vi "mainPrint.vi"(8 "Error In":errorcluster, 11 "printUDE":T1) -> (0 "Error Out":errorcluster)   [LabVIEW 2018]
uses:
  controls/printUDE.ctl
  controls/printData.ctl
  controls/serialPortEnum.ctl
panel:
  out "Boolean":bool
  in  "Print":bool
  in  "Stop":bool
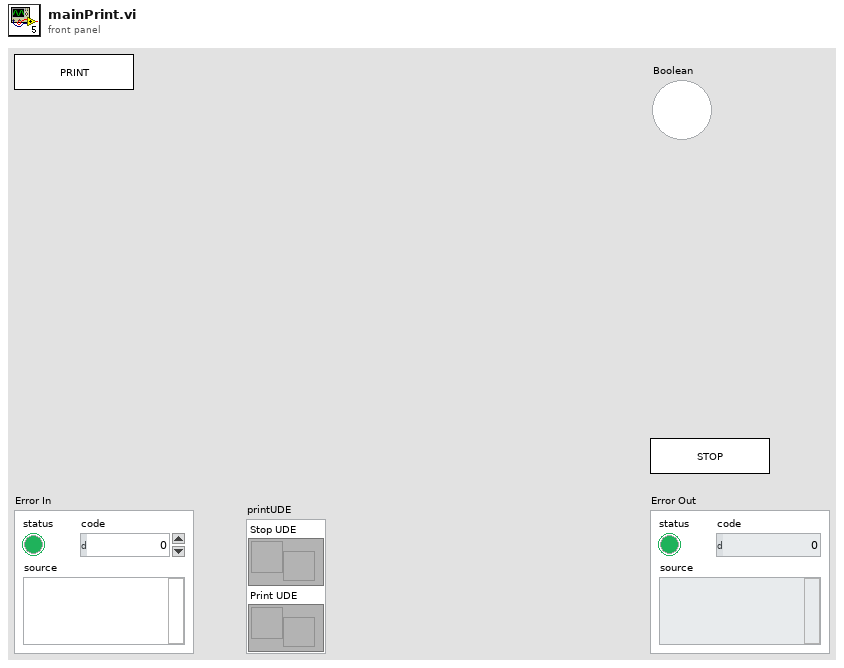
[diagram p1: front panel]
types:
  T1 = typedef "printUDE.ctl" = cluster{"Stop UDE":refnum<user-event>, "Print UDE":refnum<user-event>}
  T2 = enum32{"Invalid", "Standard", "Closed", "Hidden", "Minimized", "Maximized"}
  T3 = enum32{"invalid app kind", "Development System", "Run Time System", "Student Edition", "Embedded LabVIEW", "Evaluation", "Custom"}
  T4 = typedef "serialPortEnum.ctl" = enum16{"init", "write", "read", "close"}
  T5 = typedef "printData.ctl" = cluster{"Print Button":bool, "VISA resource name":refnum<visa-resource-name>, "Status?":bool, "Scan?":bool}
  T6 = cluster{"Core":cluster{"Current VI Reference":refnum<vi>, "Close Panel on Exit?":bool}, "printUDE":T1, "Print Data":T5, "QR":string, "Status":bool, "comPort":refnum<visa-resource-name>}
  T7 = cluster{"Current VI Reference":refnum<vi>, "Close Panel on Exit?":bool}
  T8 = typedef "pathCluster.ctl" = cluster{"src Folder Path":path, "Controller Module Path":path, "UI Module Path":path, "Model Select Module Path":path, "Barcode Printer Module Path":path, "Barcode Scanner Module Path":path, "Database Module Path":path, "Report Generation Path":path, "Simulation Path":path, "subVIs Folder Path":path, "info Folder Path":path, "config file Path":path, "cutomerLogo Path":path}
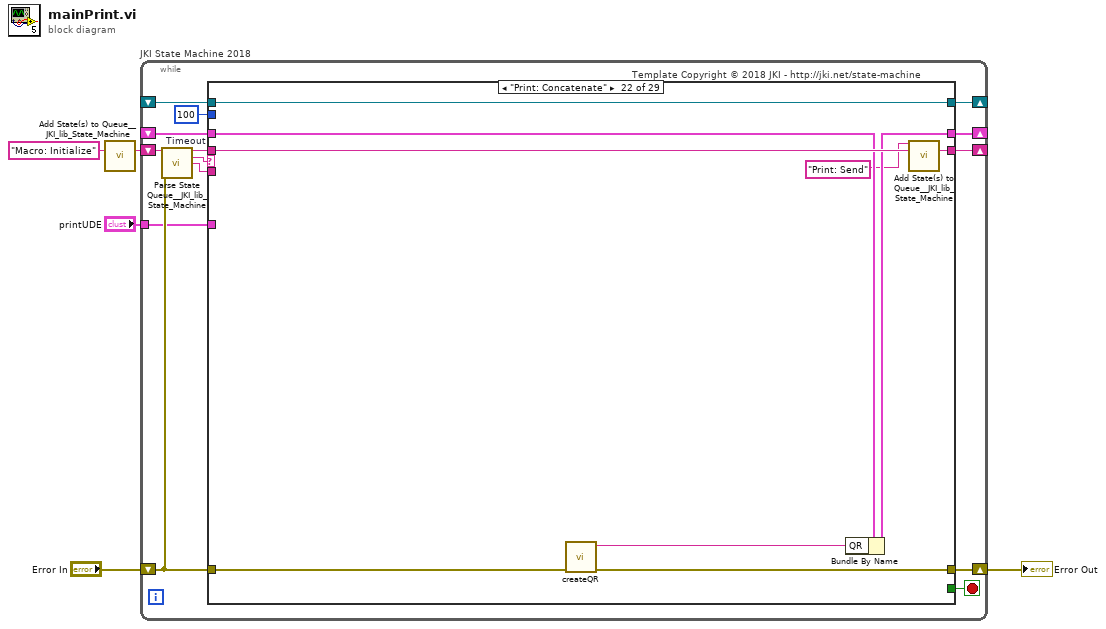
[diagram p0: block diagram]
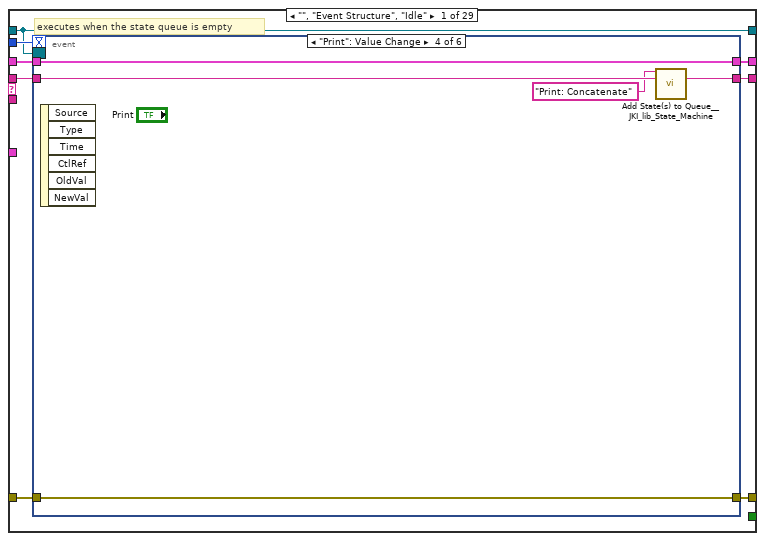
[diagram p2: hidden frame]
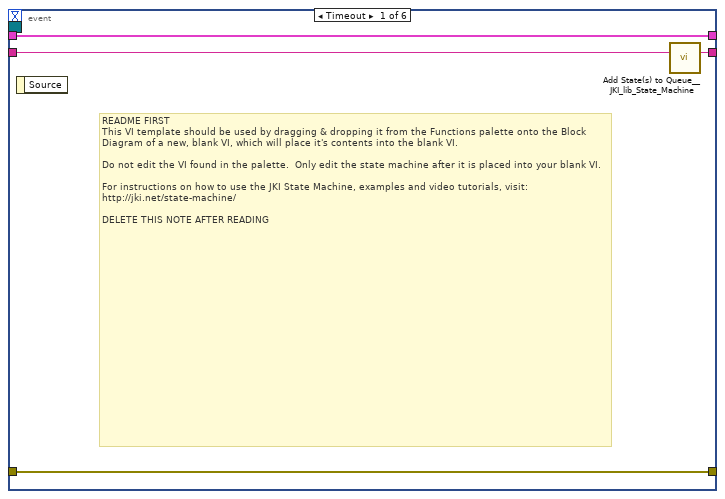
[diagram p3: hidden frame]
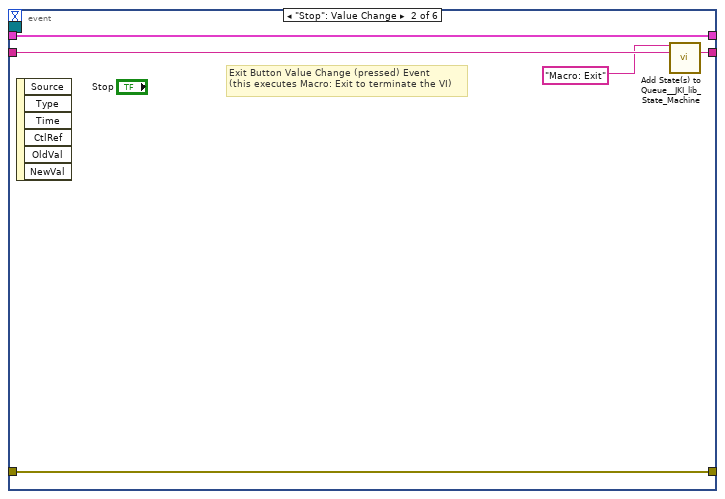
[diagram p4: hidden frame]
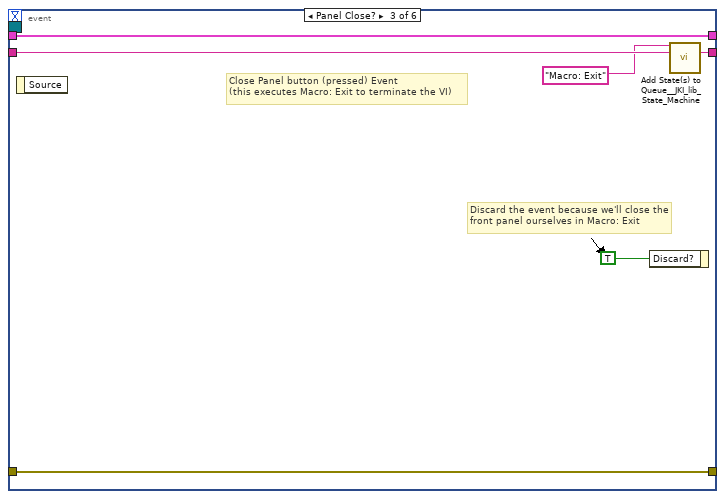
[diagram p5: hidden frame]
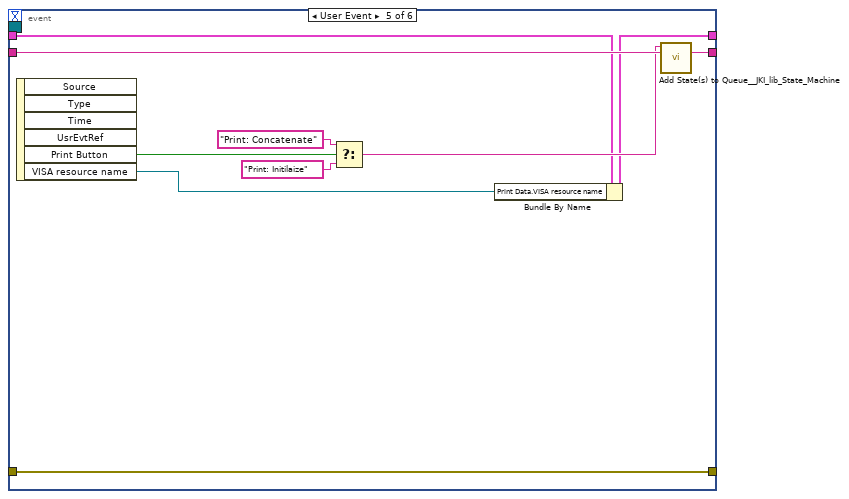
[diagram p6: hidden frame]
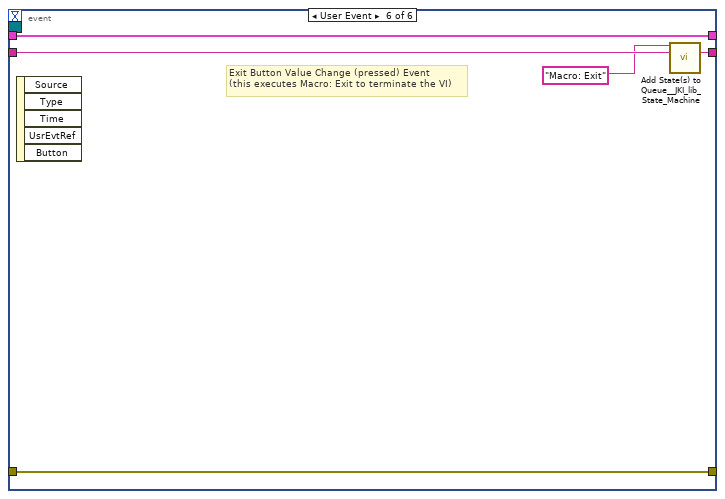
[diagram p7: hidden frame]
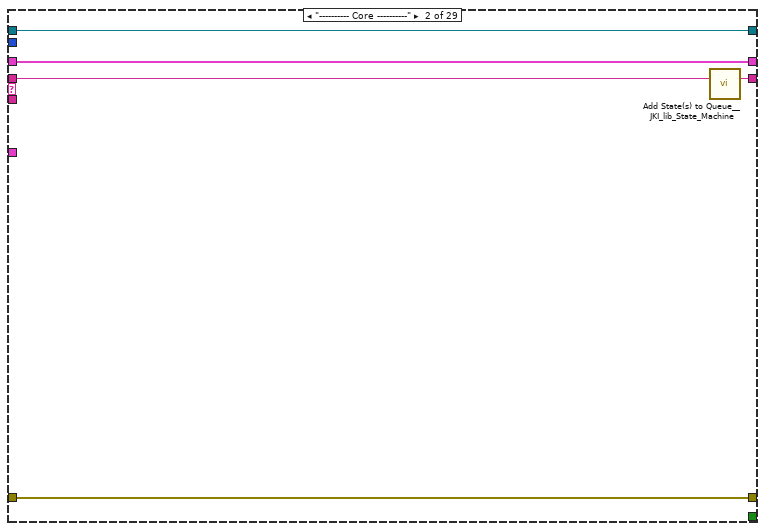
[diagram p8: hidden frame]
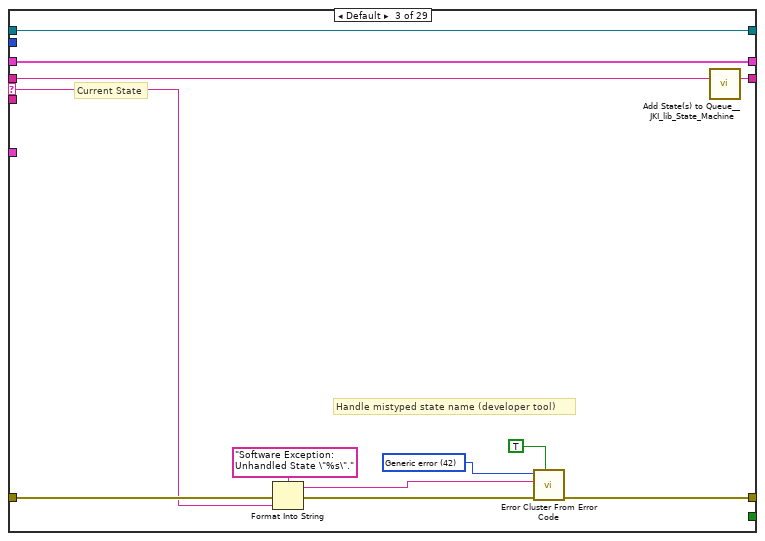
[diagram p9: hidden frame]
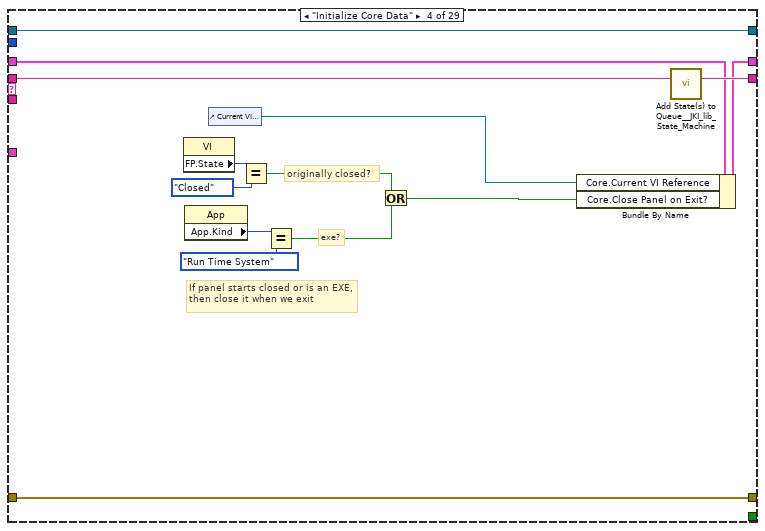
[diagram p10: hidden frame]
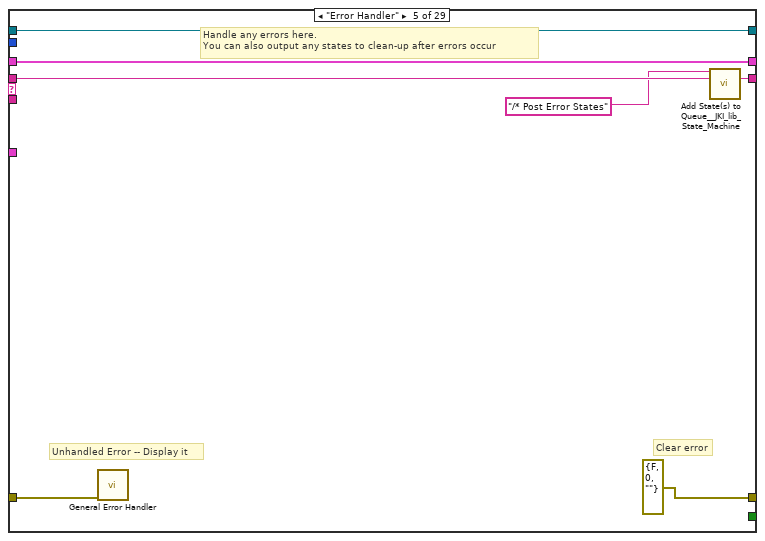
[diagram p11: hidden frame]
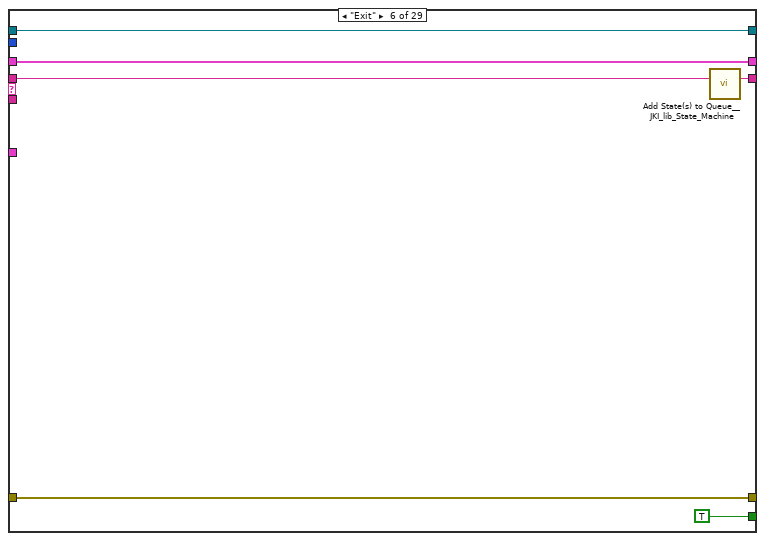
[diagram p12: hidden frame]
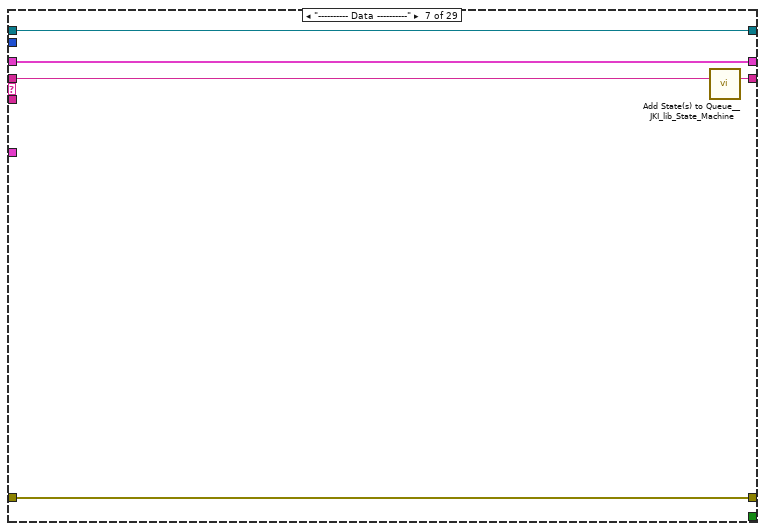
[diagram p13: hidden frame]
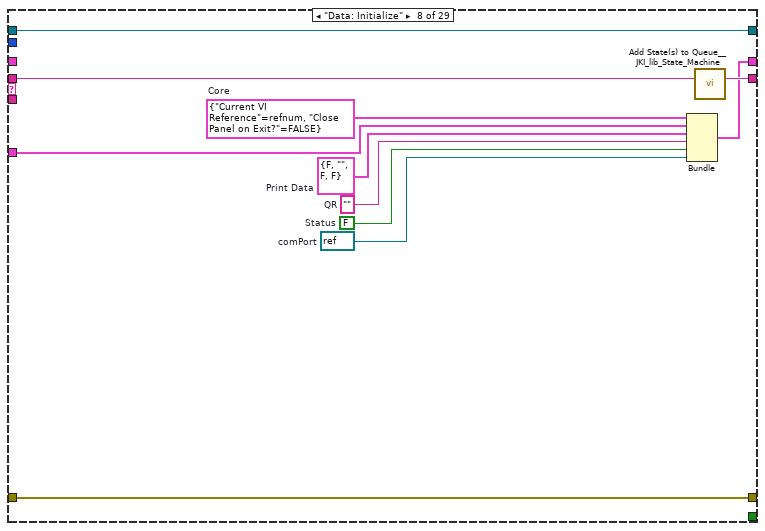
[diagram p14: hidden frame]
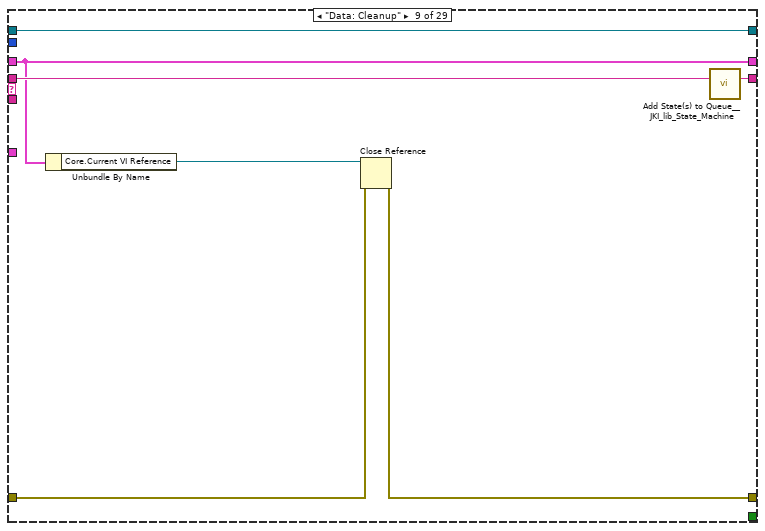
[diagram p15: hidden frame]
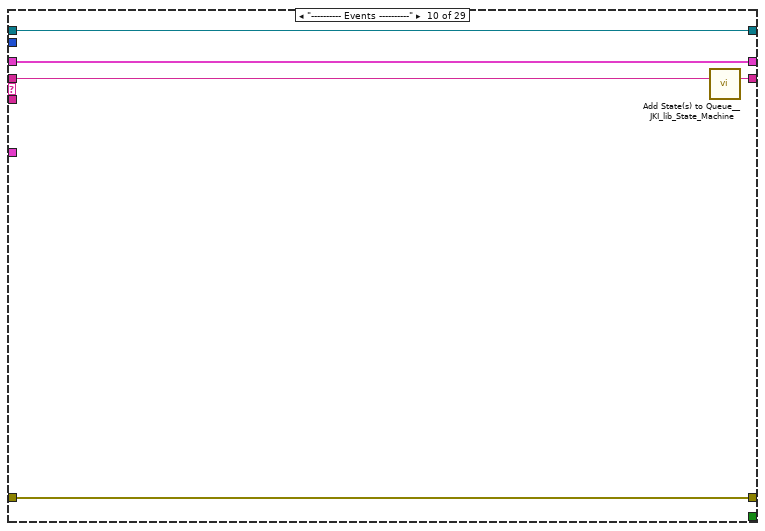
[diagram p16: hidden frame]
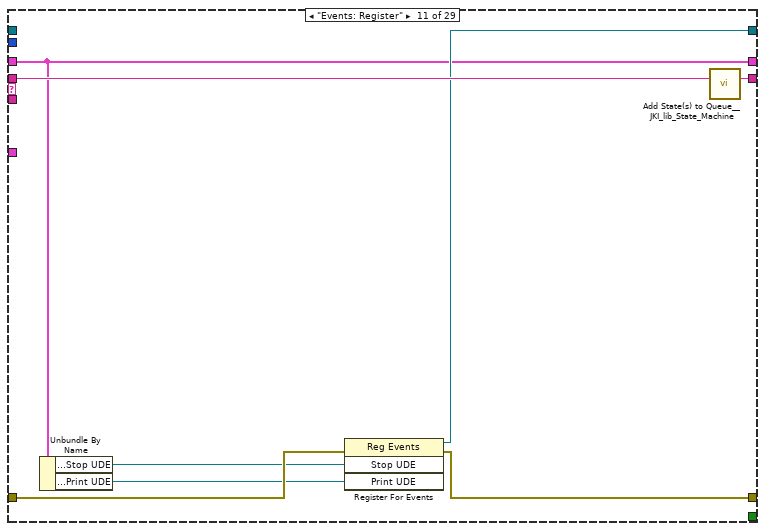
[diagram p17: hidden frame]
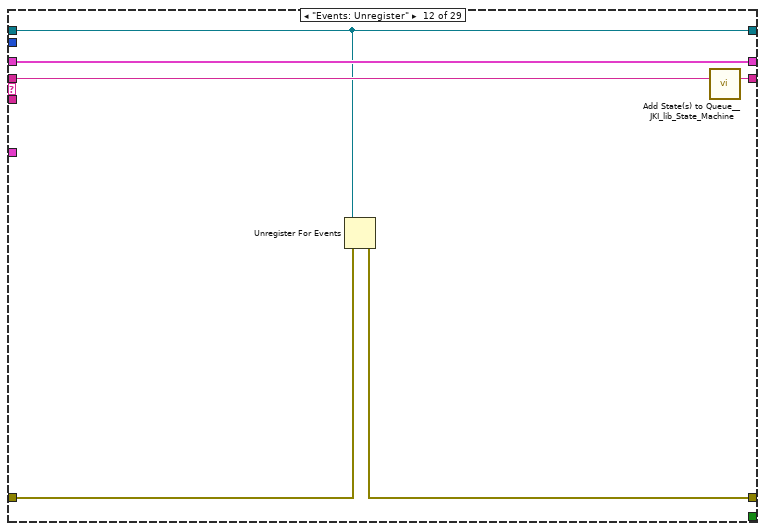
[diagram p18: hidden frame]
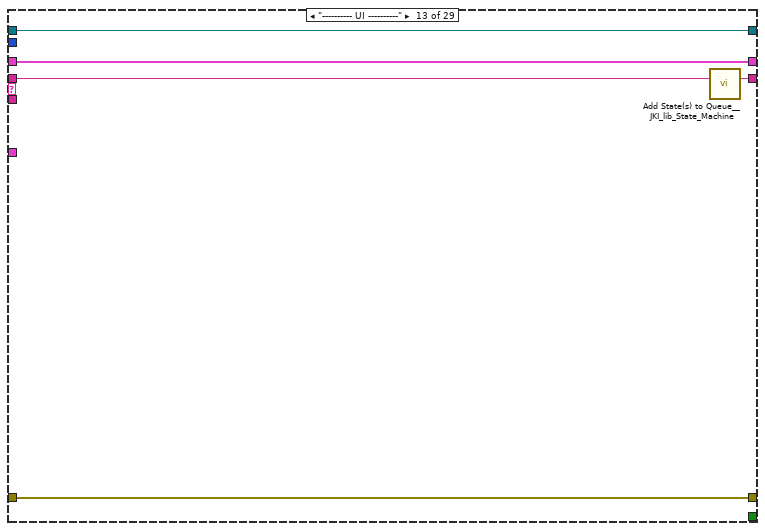
[diagram p19: hidden frame]
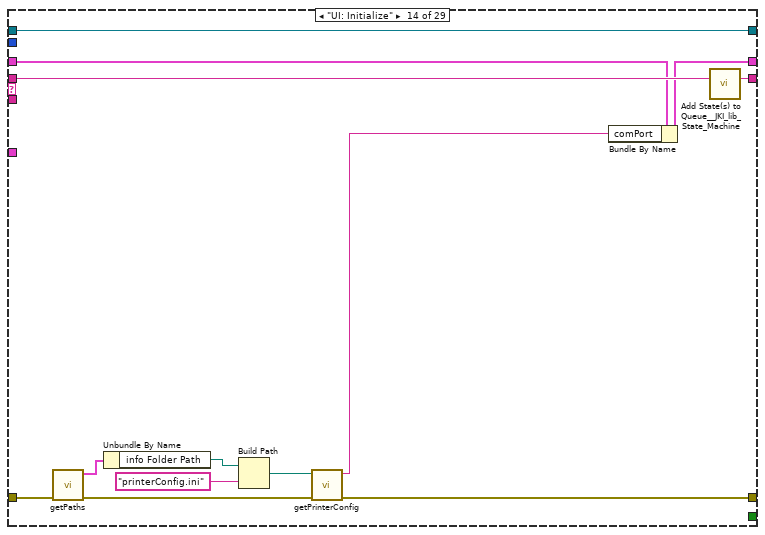
[diagram p20: hidden frame]
diagram:
  n1 = call <vilib>:"Add State(s) to Queue__JKI_lib_State_Machine.vi"("State(s) in (\"\")"="Macro: Initialize") -> ("States Out"=w5:string)  [unwired: 14 in]
  n2 = while "JKI State Machine 2018" {
    shift-right: [w12] -> _
    shift-left: _ -> [w11]
    shift-right: [w15] -> w3
    shift-left: "Error In" -> [w9]
    shift-right: [w14] -> _
    shift-left: w5 -> [w16]
    shift-right: [w8] -> _
    shift-left: _ -> [w7]
    tunnel: "printUDE" -> [w6]
    stop <- w13 stop-if-true
    w10 = 100  # Timeout
    # "Template Copyright © 2018 JKI - http://jki.net/state-machine"
    n3 = call <vilib>:"Parse State Queue__JKI_lib_State_Machine.vi"("State Queue"=w16, "Error In (no error)"=w9) -> ("Remaining States"=w18:string, "Current State"=w19:string, "Arguments"=w17:string)  [unwired: 11 in]
    n4 = case shown="\"Print: Concatenate\"" w19 {
      selector: w19 -> [_ _ w69 _ _ _ _ _ _ _ _ _ _ _ _ _ _ _ _ _ _ _ _ _ _ _ _ _ _]
      tunnel: w18 -> [w27 w67 w73 w93 w100 w106 w111 w122 w129 w134 w142 w148 w153 w166 w173 w185 w255 w261 w272 w277 w288 w297 w309 w316 w321 w333 w346 w351 w357]
      tunnel: w17 -> [_ _ _ _ _ _ _ _ _ _ _ _ _ _ w168 w179 _ _ _ _ _ _ _ _ _ _ _ _ _]
      tunnel: w11 -> [w25 w64 w71 w86 w97 w104 w108 _ w124 w131 w137 w146 w150 w156 w171 w181 w252 w258 w269 w274 w282 w292 w302 w314 w318 w324 w338 w348 w353]
      tunnel: [w24 w65 w75 w90 errorcluster {"status"=FALSE, "code"=0, "source"=""} ("error out") w103 w109 w119 w125 w132 w139 w143 w151 w158 w169 w182 w253 w259 w270 w275 w280 w293 w300 w311 w319 w329 w342 w349 w355] -> w15
      tunnel: w9 -> [w23 w65 w74 w90 w96 w103 w109 w119 w126 w132 w138 w144 w151 w163 w170 w183 w253 w259 w270 w275 w285 w294 w306 w312 w319 w330 w343 w349 w355]
      tunnel: [w26 w66 w72 w92 w99 w105 w110 w121 w128 w133 w141 w147 w152 w165 w172 w184 w254 w260 w271 w276 w287 w296 w308 w315 w320 w332 w345 w350 w356] -> w14
      tunnel: [_ _ _ _ _ TRUE _ _ _ _ _ _ _ _ _ _ _ _ _ _ _ _ _ _ _ _ _ _ _] -> w13
      tunnel: [w22 w64 w71 w91 w97 w104 w108 w120 w124 w131 w137 w146 w150 w155 w171 w181 w252 w258 w269 w274 w281 w291 w301 w314 w318 w323 w337 w348 w353] -> w12
      tunnel: w10 -> [w21 _ _ _ _ _ _ _ _ _ _ _ _ _ _ _ _ _ _ _ _ _ _ _ _ _ _ _ _]
      tunnel: [w20 w63 w68 w80 w94 w101 w107 w117 w123 w130 w140 w145 w149 w164 w167 w178 w251 w256 w262 w273 w286 w295 w307 w313 w317 w331 w344 w347 w354] -> w8
      tunnel: w7 -> [w20 w63 w68 w80 w94 w101 w107 w117 w123 w130 _ w145 w149 w164 w167 w178 w251 w256 w262 w273 w286 w295 w307 w313 w317 w331 w344 w347 w354]
      tunnel: w6 -> [_ _ _ _ _ _ _ w116 _ _ _ _ _ _ _ _ _ _ _ _ _ _ _ _ _ _ _ _ _]
      frame "", "Event Structure", "Idle" {
        # "executes when the state queue is empty"
        n5 = event shown="[3] \"Print\": Value Change" {
          selector: w20 -> [_ _ _ _ _ _]
          dyn-events: _ -> [_ _ _ _ _ _]
          timeout: w21 -> [_ _ _ _ _ _]
          tunnel: w27 -> [w31 w36 w42 w44 w54 w62]
          tunnel: [w30 w35 w41 w45 w55 w61] -> w26
          tunnel: w25 -> [w28 w33 w39 w46 w51 w59]
          tunnel: [w29 w34 w40 w47 w57 w60] -> w24
          tunnel: w23 -> [w29 w34 w40 w47 w57 w60]
          tunnel: [w28 w33 w39 w46 w50 w59] -> w22
          event Timeout {
            # "README FIRST\nThis VI template should be used by dragging & dropping it from the Functions palette onto the Block Diagram of a new, blank VI, which will place it's contents into the blank VI.\n\nDo not edit the VI found in the palette.  Only edit the state machine after it is placed into your blank VI.\n\nFor instructions on how to use the JKI State Machine, examples and video tutorials, visit:\nhttp://jki.net/state-machine/\n\nDELETE THIS NOTE AFTER READING"
            n6 = event-data() -> ()  [unwired: 1 in, 1 out]
            n7 = call <vilib>:"Add State(s) to Queue__JKI_lib_State_Machine.vi"("State(s) in (\"\")"=w31) -> ("States Out"=w30:string)  [unwired: 14 in]
          }
          event "Stop": Value Change {
            # "Exit Button Value Change (pressed) Event\n(this executes Macro: Exit to terminate the VI)"
            n8 = event-data() -> ()  [unwired: 1 in, 6 out]
            n9 = call <vilib>:"Add State(s) to Queue__JKI_lib_State_Machine.vi"("State(s) in Front (\"\")"="Macro: Exit", "State(s) in (\"\")"=w36) -> ("States Out"=w35:string)  [unwired: 13 in]
          }
          event Panel Close? {
            # "Discard the event because we'll close the front panel ourselves in Macro: Exit"
            # "Close Panel button (pressed) Event\n(this executes Macro: Exit to terminate the VI)"
            n10 = event-data() -> ()  [unwired: 1 in, 1 out]
            n11 = event-data("Discard?"=TRUE) -> ()  [unwired: 1 in, 1 out]
            n12 = call <vilib>:"Add State(s) to Queue__JKI_lib_State_Machine.vi"("State(s) in Front (\"\")"="Macro: Exit", "State(s) in (\"\")"=w42) -> ("States Out"=w41:string)  [unwired: 13 in]
          }
          event "Print": Value Change {
            n13 = event-data() -> ()  [unwired: 1 in, 6 out]
            n14 = call <vilib>:"Add State(s) to Queue__JKI_lib_State_Machine.vi"("State(s) in Front (\"\")"="Print: Concatenate" ("State(s) in Front (\"\")"), "State(s) in (\"\")"=w44) -> ("States Out"=w45:string)  [unwired: 13 in]
          }
          event User Event {
            n15 = event-data() -> ("Print Button"=w56:bool, "VISA resource name"=w49:refnum<visa-resource-name>)  [unwired: 1 in, 4 out]
            n16 = Select(t="Print: Concatenate", s=w56, f="Print: Initilaize") -> (s? t:f=w53:string)
            n17 = Bundle By Name(cluster=w51, "Print Data.VISA resource name"=w49) -> (w50:T6)
            n18 = call <vilib>:"Add State(s) to Queue__JKI_lib_State_Machine.vi"("State(s) in Front (\"\")"=w53, "State(s) in (\"\")"=w54) -> ("States Out"=w55:string)  [unwired: 13 in]
          }
          event User Event {
            # "Exit Button Value Change (pressed) Event\n(this executes Macro: Exit to terminate the VI)"
            n19 = event-data() -> ()  [unwired: 1 in, 5 out]
            n20 = call <vilib>:"Add State(s) to Queue__JKI_lib_State_Machine.vi"("State(s) in Front (\"\")"="Macro: Exit", "State(s) in (\"\")"=w62) -> ("States Out"=w61:string)  [unwired: 13 in]
          }
        }
      }
      frame "---------- Core ----------" {
        n21 = call <vilib>:"Add State(s) to Queue__JKI_lib_State_Machine.vi"("State(s) in (\"\")"=w67) -> ("States Out"=w66:string)  [unwired: 14 in]
      }
      frame Default {
        w78 = 42 items=["No error", "Argument error", "Memory is full", "Out of zone", "End of file", "File already open", "Generic file I/O error", "File not found", "File permission error", "Disk is full", "Duplicate path", "Too many files open", "System feature not enabled", "Resource file not found", "Cannot add resource", "Resource not found", "Image not found", "Image memory error", "Pen does not exist", "Config type invalid", "Config token not found", "Config parse error", "Config memory error", "Bad external code format", "Bad external code offset", "External code not present", "Null window", "Destroy window error", "Null menu", "Print aborted", "Bad print record", "Print driver error", "Windows error during printing", "Memory error during printing", "Print dialog error", "Generic print error", "Invalid device refnum", "Device not found", "Device parameter error", "Device unit error", "Cannot open device", "Device call aborted", "Generic error", "Cancelled by user", "Object ID too low", "Object ID too high", "Object not in heap", "Unknown heap", "Unknown object (invalid DefProc)", "Unknown object (DefProc not in table)", "Message out of range", "Invalid (null) method", "Unknown message", "Manager call not supported", "Bad address", "Network operation in progress", "Network operation timed out", "Connection is busy", "Network attribute not supported", "Network error", "Address in use", "System out of memory", "Connection aborted", "Connection refused", "Not connected", "Already connected", "Connection closed", "Initialization error (interapplication manager)", "Bad occurrence", "Wait on unbound occurrence handler", "Occurrence queue overflow", "Datalog type conflict", "Unused", "Unrecognized type (interapplication manager)", "Memory corrupt", "Failed to make temporary DLL", "Old CIN version", "Drag socket not found", "Failed to load drop-object", "Failed to register OLE object", "Failed to release OLE object", "Format specifier type mismatch", "Unknown format specifier", "Too few format specifiers", "Too many format specifiers", "Scan failed", "Newer CIN version", "Error converting to variant", "Runtime menu error", "Password tampered", "Variant attribute not found", "Incompatible variant data type", "Event data is not available", "Event Store is not present", "Occurrence is not found", "Event Queue is not created", "Event info is not available", "Refnum passed is NULL", "Error retrieving Class GUID", "Error retrieving CoClass GUID", "Error retrieving TypeLib GUID.", "Bad built application magic bytes.", "Specific driver is different from the specific driver associated with the Logical Name.", "There is no session opened to the class driver.", "Max Error", "MAX - Error with config objects", "MAX - Error loading configuration", "MAX - Group not supported"]
        # "Current State"
        # "Handle mistyped state name (developer tool)"
        n22 = Format Into String(format string="Software Exception: Unhandled State \"%s\"." ("message"), error in=w74, w69) -> (resulting string=w77:string, error out=w76:errorcluster)  [unwired: 1 in]
        n23 = call <vilib>:"Error Cluster From Error Code.vi"("show call chain? (False)"=TRUE, "error in (no error)"=w76, "error message (\"\")"=w77, "error code (0)"=w78) -> ("error out"=w75:errorcluster)  [unwired: 5 in]
        n24 = call <vilib>:"Add State(s) to Queue__JKI_lib_State_Machine.vi"("State(s) in (\"\")"=w73) -> ("States Out"=w72:string)  [unwired: 14 in]
      }
      frame "Initialize Core Data" {
        # "originally closed?"
        # "exe?"
        # "If panel starts closed or is an EXE, then close it when we exit"
        n25 = property class="VI"() -> ("FP.State"=w83:T2)  [unwired: 2 in, 2 out]
        n26 = property class="App"() -> ("App.Kind"=w89:T3)  [unwired: 2 in, 2 out]
        n27 = control-ref of="Current VI Reference"() -> (w84:refnum<vi>)
        n28 = Equal?(x=w83, y=T2."Closed" ("Front Panel Window:State")) -> (x = y?=w81:bool)
        n29 = Equal?(x=w89, y=T3."Run Time System" ("Application:Kind")) -> (x = y?=w87:bool)
        n30 = Or(x=w81, y=w87) -> (x .or. y?=w85:bool)
        n31 = Bundle By Name(cluster=w86, "Core.Current VI Reference"=w84, "Core.Close Panel on Exit?"=w85) -> (w91:T6)
        n32 = call <vilib>:"Add State(s) to Queue__JKI_lib_State_Machine.vi"("State(s) in (\"\")"=w93) -> ("States Out"=w92:string)  [unwired: 14 in]
      }
      frame "Error Handler" {
        # "Unhandled Error -- Display it"
        # "Handle any errors here.\nYou can also output any states to clean-up after errors occur"
        # "Clear error"
        n33 = call <vilib>:"General Error Handler.vi"("error in (no error)"=w96) -> ()  [unwired: 10 in, 5 out]
        n34 = call <vilib>:"Add State(s) to Queue__JKI_lib_State_Machine.vi"("State(s) in Front (\"\")"="/* Post Error States", "State(s) in (\"\")"=w100) -> ("States Out"=w99:string)  [unwired: 13 in]
      }
      frame "Exit" {
        n35 = call <vilib>:"Add State(s) to Queue__JKI_lib_State_Machine.vi"("State(s) in (\"\")"=w106) -> ("States Out"=w105:string)  [unwired: 14 in]
      }
      frame "---------- Data ----------" {
        n36 = call <vilib>:"Add State(s) to Queue__JKI_lib_State_Machine.vi"("State(s) in (\"\")"=w111) -> ("States Out"=w110:string)  [unwired: 14 in]
      }
      frame "Data: Initialize" {
        w112 = refnum<visa-resource-name> refnum  # comPort
        w113 = FALSE  # Status
        w114 = ""  # QR
        w115 = T5 {"Print Button"=FALSE, "VISA resource name"="", "Status?"=FALSE, "Scan?"=FALSE}  # Print Data
        w118 = T7 {"Current VI Reference"=refnum, "Close Panel on Exit?"=FALSE}  # Core
        n37 = Bundle("Core"=w118, "printUDE"=w116, "Print Data"=w115, "QR"=w114, "Status"=w113, "comPort"=w112) -> (w120:T6)  [unwired: 1 in]
        n38 = call <vilib>:"Add State(s) to Queue__JKI_lib_State_Machine.vi"("State(s) in (\"\")"=w122) -> ("States Out"=w121:string)  [unwired: 14 in]
      }
      frame "Data: Cleanup" {
        n39 = Unbundle By Name(w124) -> ("Core.Current VI Reference"=w127:refnum<vi>)
        n40 = Close Reference(reference=w127, error in (no error)=w126) -> (error out=w125:errorcluster)
        n41 = call <vilib>:"Add State(s) to Queue__JKI_lib_State_Machine.vi"("State(s) in (\"\")"=w129) -> ("States Out"=w128:string)  [unwired: 14 in]
      }
      frame "---------- Events ----------" {
        n42 = call <vilib>:"Add State(s) to Queue__JKI_lib_State_Machine.vi"("State(s) in (\"\")"=w134) -> ("States Out"=w133:string)  [unwired: 14 in]
      }
      frame "Events: Register" {
        n43 = Unbundle By Name(w137) -> ("printUDE.Stop UDE"=w136:refnum<user-event>, "printUDE.Print UDE"=w135:refnum<user-event>)
        n44 = register-events(error in=w138, w136, w135) -> (reference out=w140:refnum<event-registration>, error out=w139:errorcluster)  [unwired: 1 in]
        n45 = call <vilib>:"Add State(s) to Queue__JKI_lib_State_Machine.vi"("State(s) in (\"\")"=w142) -> ("States Out"=w141:string)  [unwired: 14 in]
      }
      frame "Events: Unregister" {
        n46 = Unregister For Events(event registration refnum=w145, error in=w144) -> (error out=w143:errorcluster)
        n47 = call <vilib>:"Add State(s) to Queue__JKI_lib_State_Machine.vi"("State(s) in (\"\")"=w148) -> ("States Out"=w147:string)  [unwired: 14 in]
      }
      frame "---------- UI ----------" {
        n48 = call <vilib>:"Add State(s) to Queue__JKI_lib_State_Machine.vi"("State(s) in (\"\")"=w153) -> ("States Out"=w152:string)  [unwired: 14 in]
      }
      frame "UI: Initialize" {
        n49 = call "getPaths.vi"("Error In"=w163) -> ("Error Out"=w159:errorcluster, "Application Path Cluster"=w162:T8)  [unwired: 9 in]
        n50 = Unbundle By Name(w162) -> ("info Folder Path"=w161:path)
        n51 = Build Path(base path=w161, name or relative path="printerConfig.ini") -> (appended path=w157:path)
        n52 = call "getPrinterConfig.vi"("Error In"=w159, "Config File Path"=w157) -> ("Error Out"=w158:errorcluster, "comPort"=w154:string)  [unwired: 8 in]
        n53 = Bundle By Name(cluster=w156, "comPort"=w154) -> (w155:T6)
        n54 = call <vilib>:"Add State(s) to Queue__JKI_lib_State_Machine.vi"("State(s) in (\"\")"=w166) -> ("States Out"=w165:string)  [unwired: 14 in]
      }
      frame "UI: Cursor Set" {
        # "Argument"
        n55 = case shown="\"Idle\", Default" w168 {
          tunnel: w170 -> [w175 w177]
          tunnel: [w174 w176] -> w169
          frame "Idle", Default {
            n56 = call <vilib>:"Unset Busy.vi"("error in (no error)"=w175) -> ("error out"=w174:errorcluster)  [unwired: 10 in]
          }
          frame "Busy" {
            n57 = call <vilib>:"Set Busy.vi"("error in (no error)"=w177) -> ("error out"=w176:errorcluster)  [unwired: 9 in, 1 out]
          }
        }
        n58 = call <vilib>:"Add State(s) to Queue__JKI_lib_State_Machine.vi"("State(s) in (\"\")"=w173) -> ("States Out"=w172:string)  [unwired: 14 in]
      }
      frame "UI: Front Panel State" {
        # "Argument"
        n59 = Unbundle By Name(w181) -> ("Core.Current VI Reference"=w180:refnum<vi>)
        n60 = case shown="\"Minimize\", \"Minimized\"" w179 {
          tunnel: w183 -> [w191 w206 w217 w230 w243]
          tunnel: [w193 w207 w219 w232 w245] -> w182
          tunnel: w180 -> [w192 w204 w218 w231 w244]
          frame "Open", "Standard", Default {
            w186 = T2."Standard" ("State")
            n61 = property class="VI"(reference=w192, error in=w191) -> (reference out=w189:refnum<vi>, error out=w190:errorcluster, "FP.State"=w188:T2)
            n62 = Not Equal?(x=w188, y=w186) -> (x != y?=w187:bool)
            n63 = case shown="True" w187 {
              tunnel: [w197 w199] -> w193
              tunnel: w190 -> [w196 w199]
              tunnel: w189 -> [w195 _]
              tunnel: w186 -> [w194 _]
              frame True {
                n64 = invoke class="VI" method="FP.Open"(reference=w195, error in=w196, "Activate"=TRUE, "State"=w194) -> (error out=w197:errorcluster)  [unwired: 1 in, 4 out]
              }
              frame False {
              }
            }
          }
          frame "Close", "Closed" {
            n65 = property class="VI"(reference=w204, error in=w206) -> (reference out=w203:refnum<vi>, error out=w205:errorcluster, "FP.State"=w201:T2)
            n66 = Not Equal?(x=w201, y=T2."Closed" ("Front Panel Window:State")) -> (x != y?=w200:bool)
            n67 = case shown="True" w200 {
              tunnel: [w208 w211] -> w207
              tunnel: w205 -> [w208 w210]
              tunnel: w203 -> [_ w209]
              frame False {
              }
              frame True {
                n68 = invoke class="VI" method="FP.Close"(reference=w209, error in=w210) -> (error out=w211:errorcluster)  [unwired: 1 in, 2 out]
              }
            }
          }
          frame "Hidden", "Hide" {
            w212 = T2."Hidden" ("State")
            n69 = property class="VI"(reference=w218, error in=w217) -> (reference out=w215:refnum<vi>, error out=w216:errorcluster, "FP.State"=w214:T2)
            n70 = Not Equal?(x=w214, y=w212) -> (x != y?=w213:bool)
            n71 = case shown="True" w213 {
              tunnel: [w223 w224] -> w219
              tunnel: w216 -> [w222 w224]
              tunnel: w215 -> [w221 _]
              tunnel: w212 -> [w220 _]
              frame True {
                n72 = invoke class="VI" method="FP.Open"(reference=w221, error in=w222, "State"=w220) -> (error out=w223:errorcluster)  [unwired: 2 in, 4 out]
              }
              frame False {
              }
            }
          }
          frame "Minimize", "Minimized" {
            w225 = T2."Minimized" ("State")
            n73 = property class="VI"(reference=w231, error in=w230) -> (reference out=w228:refnum<vi>, error out=w229:errorcluster, "FP.State"=w227:T2)
            n74 = Not Equal?(x=w227, y=w225) -> (x != y?=w226:bool)
            n75 = case shown="True" w226 {
              tunnel: [w236 w237] -> w232
              tunnel: w229 -> [w235 w237]
              tunnel: w228 -> [w234 _]
              tunnel: w225 -> [w233 _]
              frame True {
                n76 = invoke class="VI" method="FP.Open"(reference=w234, error in=w235, "State"=w233) -> (error out=w236:errorcluster)  [unwired: 2 in, 4 out]
              }
              frame False {
              }
            }
          }
          frame "Maximize", "Maximized" {
            w238 = T2."Maximized" ("State")
            n77 = property class="VI"(reference=w244, error in=w243) -> (reference out=w241:refnum<vi>, error out=w242:errorcluster, "FP.State"=w240:T2)
            n78 = Not Equal?(x=w240, y=w238) -> (x != y?=w239:bool)
            n79 = case shown="True" w239 {
              tunnel: [w249 w250] -> w245
              tunnel: w242 -> [w248 w250]
              tunnel: w241 -> [w247 _]
              tunnel: w238 -> [w246 _]
              frame True {
                n80 = invoke class="VI" method="FP.Open"(reference=w247, error in=w248, "State"=w246) -> (error out=w249:errorcluster)  [unwired: 2 in, 4 out]
              }
              frame False {
              }
            }
          }
        }
        n81 = call <vilib>:"Add State(s) to Queue__JKI_lib_State_Machine.vi"("State(s) in (\"\")"=w185) -> ("States Out"=w184:string)  [unwired: 14 in]
      }
      frame "---------- Macro ----------" {
        n82 = call <vilib>:"Add State(s) to Queue__JKI_lib_State_Machine.vi"("State(s) in (\"\")"=w255) -> ("States Out"=w254:string)  [unwired: 14 in]
      }
      frame "Macro: Initialize" {
        n83 = call <vilib>:"Add State(s) to Queue__JKI_lib_State_Machine.vi"("State(s) in Front (\"\")"="Data: Initialize\nInitialize Core Data\nEvents: Register\nUI: Initialize\nPrint: Initilaize\nUI: Front Panel State >> Open", "State(s) in (\"\")"=w261) -> ("States Out"=w260:string)  [unwired: 13 in]
      }
      frame "Macro: Exit" {
        n84 = Unbundle By Name(w269) -> ("Core.Close Panel on Exit?"=w268:bool)
        n85 = Select(t="UI: Front Panel State >> Close", s=w268, f="") -> (s? t:f=w265:string)
        n86 = call <vilib>:"Add State(s) to Queue__JKI_lib_State_Machine.vi"("State(s) in (\"\")"=w265, "State(s) at Back (\"\")"="Print: Close\nData: Cleanup\nEvents: Unregister\nExit") -> ("States Out"=w263:string)  [unwired: 13 in]
        n87 = call <vilib>:"Add State(s) to Queue__JKI_lib_State_Machine.vi"("State(s) in Front (\"\")"=w263, "State(s) in (\"\")"=w272) -> ("States Out"=w271:string)  [unwired: 13 in]
      }
      frame "---------- Print ----------" {
        n88 = call <vilib>:"Add State(s) to Queue__JKI_lib_State_Machine.vi"("State(s) in (\"\")"=w277) -> ("States Out"=w276:string)  [unwired: 14 in]
      }
      frame "Print: Initilaize" {
        n89 = Unbundle By Name(w282) -> ("Print Data.VISA resource name"=w283:refnum<visa-resource-name>)
        n90 = call "serialDriver.vi"("Serial Port Enum"=serialPortEnum."init", "Error In"=w285, "VISA resource name"=w283) -> ("Error Out"=w280:errorcluster)  [unwired: 7 in, 1 out]
        n91 = Unbundle By Name(w280) -> ("status"=w279:bool)
        n92 = Not(x=w279) -> (.not. x?=w278:bool)
        n93 = Bundle By Name(cluster=w282, "Status"=w278) -> (w281:T6)
        n94 = call <vilib>:"Add State(s) to Queue__JKI_lib_State_Machine.vi"("State(s) in (\"\")"=w288) -> ("States Out"=w287:string)  [unwired: 14 in]
      }
      frame "Print: Concatenate" {
        n95 = call "createQR.vi"("Error In"=w294) -> ("Error Out"=w293:errorcluster, "QR"=w290:string)  [unwired: 9 in]
        n96 = Bundle By Name(cluster=w292, "QR"=w290) -> (w291:T6)
        n97 = call <vilib>:"Add State(s) to Queue__JKI_lib_State_Machine.vi"("State(s) in Front (\"\")"="Print: Send" ("State(s) in Front (\"\")"), "State(s) in (\"\")"=w297) -> ("States Out"=w296:string)  [unwired: 13 in]
      }
      frame "Print: Send" {
        n98 = Unbundle By Name(w302) -> ("QR"=w304:string)
        n99 = call "serialDriver.vi"("Serial Port Enum"=serialPortEnum."write", "Error In"=w306, "Value In"=w304) -> ("Error Out"=w300:errorcluster)  [unwired: 7 in, 1 out]
        n100 = Unbundle By Name(w300) -> ("status"=w299:bool)
        n101 = Not(x=w299) -> (.not. x?=w298:bool)
        n102 = Bundle By Name(cluster=w302, "Status"=w298) -> (w301:T6)
        n103 = call <vilib>:"Add State(s) to Queue__JKI_lib_State_Machine.vi"("State(s) in Front (\"\")"="Generate: Scan" ("State(s) in Front (\"\")"), "State(s) in (\"\")"=w309) -> ("States Out"=w308:string)  [unwired: 13 in]
      }
      frame "Print: Close" {
        n104 = call "serialDriver.vi"("Serial Port Enum"=serialPortEnum."close", "Error In"=w312) -> ("Error Out"=w311:errorcluster)  [unwired: 8 in, 1 out]
        n105 = call <vilib>:"Add State(s) to Queue__JKI_lib_State_Machine.vi"("State(s) in (\"\")"=w316) -> ("States Out"=w315:string)  [unwired: 14 in]
      }
      frame "---------- Generate ----------" {
        n106 = call <vilib>:"Add State(s) to Queue__JKI_lib_State_Machine.vi"("State(s) in (\"\")"=w321) -> ("States Out"=w320:string)  [unwired: 14 in]
      }
      frame "Generate: Status" {
        n107 = Unbundle By Name(w324) -> ("Status"=w325:bool, "printUDE.Print UDE"=w328:refnum<user-event>)
        n108 = Bundle By Name(cluster=T5 {"Print Button"=FALSE, "VISA resource name"="", "Status?"=FALSE, "Scan?"=FALSE} ("event data"), "Status?"=w325) -> (w326:T5)
        n109 = Generate User Event(user event=w328, event data cluster=w326, error in=w330) -> (user event out=w322:refnum<user-event>, error out=w329:errorcluster)  [unwired: 1 in]
        n110 = Bundle By Name(cluster=w324, "printUDE.Print UDE"=w322) -> (w323:T6)
        n111 = call <vilib>:"Add State(s) to Queue__JKI_lib_State_Machine.vi"("State(s) in (\"\")"=w333) -> ("States Out"=w332:string)  [unwired: 14 in]
      }
      frame "Generate: Scan" {
        n112 = Unbundle By Name(w338) -> ("Status"=w334:bool, "printUDE.Print UDE"=w341:refnum<user-event>)
        n113 = Bundle By Name(cluster=T5 {"Print Button"=FALSE, "VISA resource name"="", "Status?"=FALSE, "Scan?"=FALSE} ("event data"), "Status?"=w334, "Scan?"=w334) -> (w339:T5)
        n114 = Generate User Event(user event=w341, event data cluster=w339, error in=w343) -> (user event out=w336:refnum<user-event>, error out=w342:errorcluster)  [unwired: 1 in]
        n115 = Bundle By Name(cluster=w338, "printUDE.Print UDE"=w336) -> (w337:T6)
        n116 = call <vilib>:"Add State(s) to Queue__JKI_lib_State_Machine.vi"("State(s) in Front (\"\")"="Generate: Scan" ("State(s) in Front (\"\")"), "State(s) in (\"\")"=w346) -> ("States Out"=w345:string)  [unwired: 13 in]
      }
      frame "---------- Display ----------" {
        n117 = call <vilib>:"Add State(s) to Queue__JKI_lib_State_Machine.vi"("State(s) in (\"\")"=w351) -> ("States Out"=w350:string)  [unwired: 14 in]
      }
      frame "Display: Status" {
        n118 = Unbundle By Name(w353) -> ("Status"=→"Boolean":bool)
        n119 = call <vilib>:"Add State(s) to Queue__JKI_lib_State_Machine.vi"("State(s) in (\"\")"=w357) -> ("States Out"=w356:string)  [unwired: 14 in]
      }
    }
  }
  "Error Out" <- w3
